vi "Matlab clear and close all.vi"(8 "error in (no error)":errorcluster) -> (0 "error out":errorcluster)   [LabVIEW 2020]
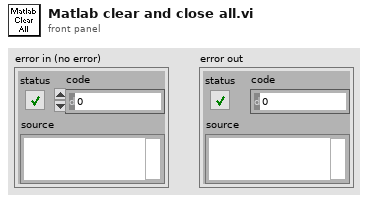
[diagram p1: front panel]
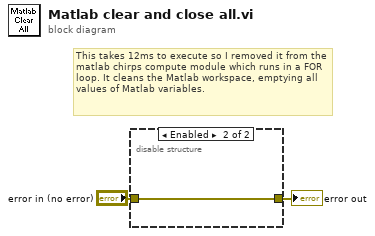
[diagram p0: block diagram]
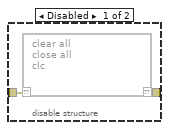
[diagram p2: hidden frame]
diagram:
  # "This takes 12ms to execute so I removed it from the matlab chirps compute module which runs in a FOR loop. It cleans the Matlab workspace, emptying all values of Matlab variables."
  n1 = disable-structure shown="Enabled" {
    disable-tunnel: [w4 w5] -> w2
    disable-tunnel: "error in (no error)" -> [w3 w5]
    frame Disabled {
      n2 = script code="clear all\nclose all\nclc" ("Script Node")("??"=w3) -> ("??"=w4:errorcluster)
    }
    frame Enabled {
    }
  }
  "error out" <- w2
